vi "Mcp2210 Get Gpio Config.vi"(6 "error in (no error)":errorcluster, 8 "Chip Setting Selection":T2(ring), 9 "handle":i32) -> (0 "error out":errorcluster, 2 "GPIO CFG":T1, 3 "handle out":i32)   [LabVIEW 2015, in "mcp2210.lvlib"]
doc: "Provides the current GPIO configuration or the power-up default (NVRAM) GPIO configuration.\nParameters:\nInputs:\n- IntPtr handle - The device handle. Cannot be NULL.\n- unsigned char cfgSelector - current/power-up chip setting selection. Valid values are:\n- M_MCP2210_VM_CONFIG: designates current chip setting (Volatile\nMemory)\n- M_MCP2210_NVRAM_CONFIG: designates power-up chip setting (NVRAM)\nOutputs:\n- array<Byte>^ pGpioPinDes - GPIO Pin Designation array. Cannot be NULL.\nArray length must be M_MCP2210_GPIO_NR.\nValid values for pin designation are:\n- M_MCP2210_PIN_DES_GPIO\n- M_MCP2210_PIN_DES_CS\n- M_MCP2210_PIN_DES_FN\n- unsigned int %pdfltGpioOutput - GPIO pin output values.\n- unsigned int %pdfltGpioDir - GPIO pin direction.\n- unsigned char %prmtWkupEn - remote wake-up setting. Valid values:\n- M_MCP2210_REMOTE_WAKEUP_ENABLED\n- M_MCP2210_REMOTE_WAKEUP_DISABLED\n- unsigned char %pintPinMd - interrupt pulse count mode. Valid values are:\n- M_MCP2210_INT_MD_CNT_HIGH_PULSES\n- M_MCP2210_INT_MD_CNT_LOW_PULSES\n- M_MCP2210_INT_MD_CNT_RISING_EDGES\n- M_MCP2210_INT_MD_CNT_FALLING_EDGES\n- M_MCP2210_INT_MD_CNT_NONE\n- unsigned char %pspiBusRelEn - SPI Bus Release option. Valid values are:\n- M_MCP2210_SPI_BUS_RELEASE_ENABLED\n- M_MCP2210_SPI_BUS_RELEASE_DISABLED\nReturns:\n- 0 for success: M_E_SUCCESS\n- negative error code: M_E_ERR_NULL, M_E_ERR_INVALID_HANDLE_VALUE\nM_E_ERR_UNKOWN_ERROR, M_E_ERR_INVALID_PARAMETER\nM_E_ERR_HID_TIMEOUT, M_E_ERR_HID_RW_FILEIO\nM_E_ERR_CMD_ECHO, M_E_ERR_CMD_FAILED\n\nMCP2210_DLL_UM_API int __stdcall Mcp2210_GetGpioConfig(void *handle, unsigned char cfgSelector, unsigned char *pGpioPinDes, unsigned int *pdfltGpioOutput,\n unsigned int *pdfltGpioDir, unsigned char *prmtWkupEn, unsigned char *pintPinMd, unsigned char *pspiBusRelEn);"
uses:
  <userlib>/mcp2210/mcp2210.lvlib
  <userlib>/mcp2210/mcp2210_dll_um_x86.dll
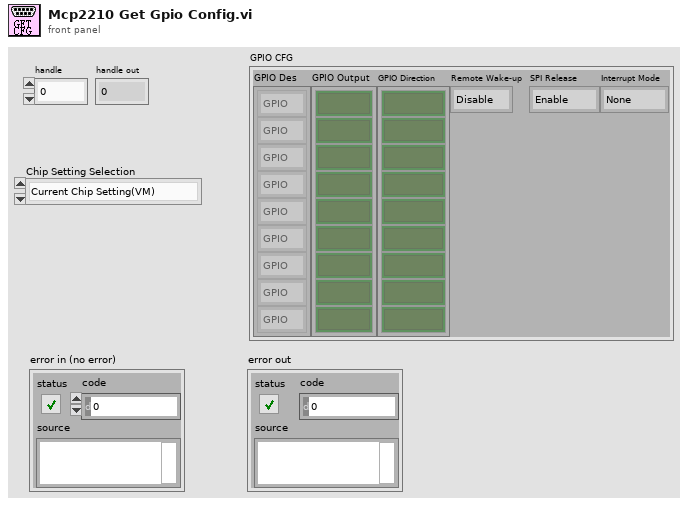
[diagram p1: front panel]
types:
  T1 = cluster{"GPIO Des":enum8{"GPIO", "CS", "Dedicated"}[], "GPIO Output":bool[], "GPIO Direction":bool[], "Remote Wake-up":enum16{"Disable", "Enable"}, "SPI Release":enum16{"Enable", "Disable"}, "Interrupt Mode":enum16{"None", "Falling", "Rising", "Low", "High"}}
  T2 = enum8{"Current Chip Setting(VM)", "Power-up Chip Setting(NVRAM)"}
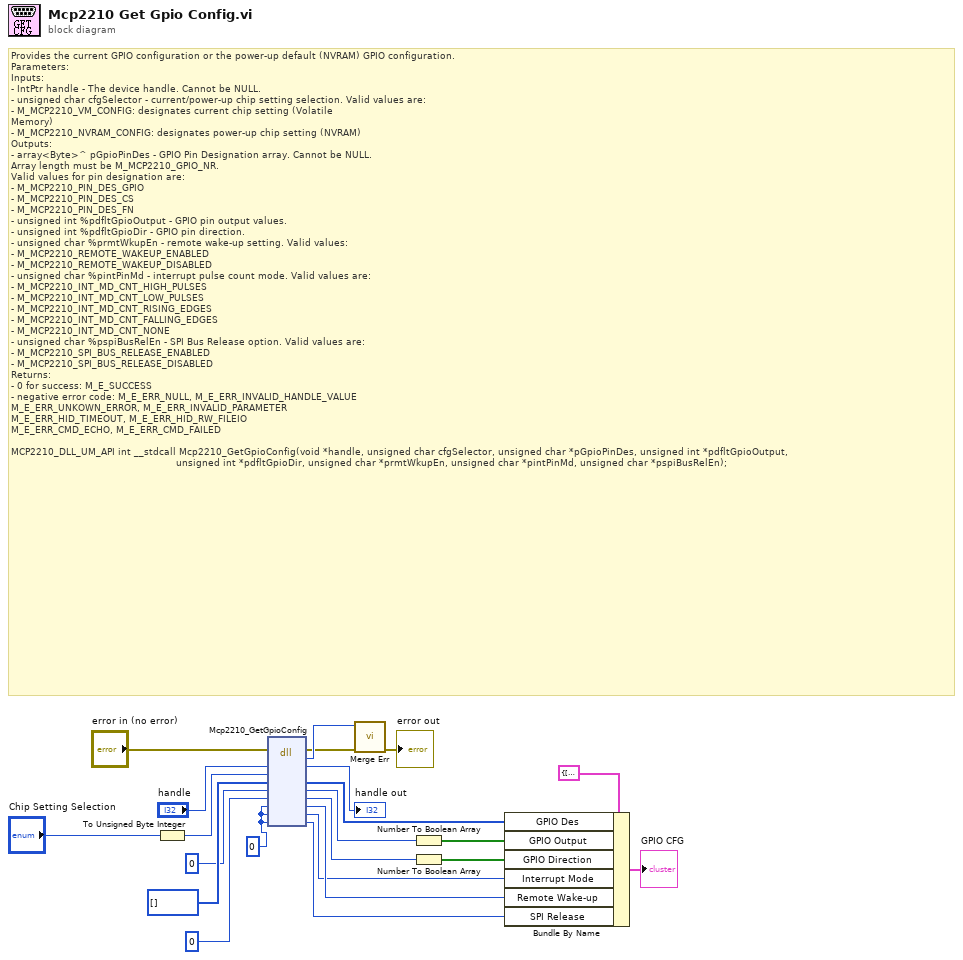
[diagram p0: block diagram]
diagram:
  w1 = u8 0 ("pdfltGpioDir")
  # "Provides the current GPIO configuration or the power-up default (NVRAM) GPIO configuration.\nParameters:\nInputs:\n- IntPtr handle - The device handle. Cannot be NULL.\n- unsigned char cfgSelector - current/power-up chip setting selection. Valid values are:\n- M_MCP2210_VM_CONFIG: designates current chip setting (Volatile\nMemory)\n- M_MCP2210_NVRAM_CONFIG: designates power-up chip setting (NVRAM)\nOutputs:\n- array<Byte>^ pGpioPinDes - GPIO Pin Designation array. Cannot be NULL.\nArray length must be M_MCP2210_GPIO_NR.\nValid values for pin designation are:\n- M_MCP2210_PIN_DES_GPIO\n- M_MCP2210_PIN_DES_CS\n- M_MCP2210_PIN_DES_FN\n- unsigned int %pdfltGpioOutput - GPIO pin output values.\n- unsigned int %pdfltGpioDir - GPIO pin direction.\n- unsigned char %prmtWkupEn - remote wake-up setting. Valid values:\n- M_MCP2210_REMOTE_WAKEUP_ENABLED\n- M_MCP2210_REMOTE_WAKEUP_DISABLED\n- unsigned char %pintPinMd - interrupt pulse count mode. Valid values are:\n- M_MCP2210_INT_MD_CNT_HIGH_PULSES\n- M_MCP2210_INT_MD_CNT_LOW_PULSES\n- M_MCP2210_INT_MD_CNT_RISING_EDGES\n- M_MCP2210_INT_MD_CNT_FALLING_EDGES\n- M_MCP2210_INT_MD_CNT_NONE\n- unsigned char %pspiBusRelEn - SPI Bus Release option. Valid values are:\n- M_MCP2210_SPI_BUS_RELEASE_ENABLED\n- M_MCP2210_SPI_BUS_RELEASE_DISABLED\nReturns:\n- 0 for success: M_E_SUCCESS\n- negative error code: M_E_ERR_NULL, M_E_ERR_INVALID_HANDLE_VALUE\nM_E_ERR_UNKOWN_ERROR, M_E_ERR_INVALID_PARAMETER\nM_E_ERR_HID_TIMEOUT, M_E_ERR_HID_RW_FILEIO\nM_E_ERR_CMD_ECHO, M_E_ERR_CMD_FAILED\n\nMCP2210_DLL_UM_API int __stdcall Mcp2210_GetGpioConfig(void *handle, unsigned char cfgSelector, unsigned char *pGpioPinDes, unsigned int *pdfltGpioOutput,\n                                                       unsigned int *pdfltGpioDir, unsigned char *prmtWkupEn, unsigned char *pintPinMd, unsigned char *pspiBusRelEn);"
  n1 = To Unsigned Byte Integer(number="Chip Setting Selection") -> (unsigned 8bit integer=w18:u8)
  n2 = dll-call lib="D:/LabVIEW 2015/user.lib/mcp2210/mcp2210_dll_um_x86.*" fn="Mcp2210_GetGpioConfig"(error in="error in (no error)", "handle"="handle", "cfgSelector"=w18, "pGpioPinDes"=u8[] [], "pdfltGpioOutput"=u32 0, "pdfltGpioDir"=u32 0, "prmtWkupEn"=w1, "pintPinMd"=w1, "pspiBusRelEn"=w1) -> (error out=w16:errorcluster, "return type"=w17:i32, "handle"=→"handle out":i32, "pGpioPinDes"=w13:u8[], "pdfltGpioOutput"=w12:u32, "pdfltGpioDir"=w10:u32, "prmtWkupEn"=w5:u8, "pintPinMd"=w2:u8, "pspiBusRelEn"=w3:u8)  [unwired: 3 in, 1 out]
  n3 = call <userlib>:"Merge Err.vi"("error in (no error)"=w16, "return type"=w17) -> ("error out"=→"error out":errorcluster)  [unwired: 9 in]
  n4 = Number To Boolean Array(number=w12) -> (Boolean array=w11:bool[])
  n5 = Number To Boolean Array(number=w10) -> (Boolean array=w8:bool[])
  n6 = Bundle By Name(cluster=T1 {"GPIO Des"=[], "GPIO Output"=[], "GPIO Direction"=[], "Remote Wake-up"=enum."Disable", "SPI Release"=enum."Enable", "Interrupt Mode"=enum."None"} ("GPIO CFG"), "GPIO Des"=w13, "GPIO Output"=w11, "GPIO Direction"=w8, "Interrupt Mode"=w2, "Remote Wake-up"=w5, "SPI Release"=w3) -> (→"GPIO CFG":T1)
